vi "setMode.vi"(8 "error in (no error)":errorcluster, 10 "mode":enum16{"current", "voltage"}[](array[ring]), 11 "ethernetSupply in":refnum<class "ethernetSupply.lvclass">) -> (0 "error out":errorcluster, 3 "ethernetSupply out":refnum<class "ethernetSupply.lvclass">)   [LabVIEW 2011, in "Tools.lvlib" / "DatabaseHelpers.lvlib" / "ethernetSupply.lvclass"]
uses:
  ethernetSupply.lvclass
  ethernetSupply.lvclass/ethernetSupply.ctl
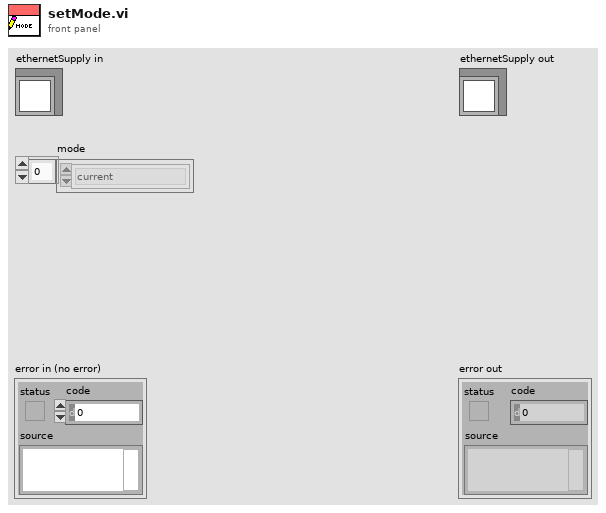
[diagram p1: front panel]
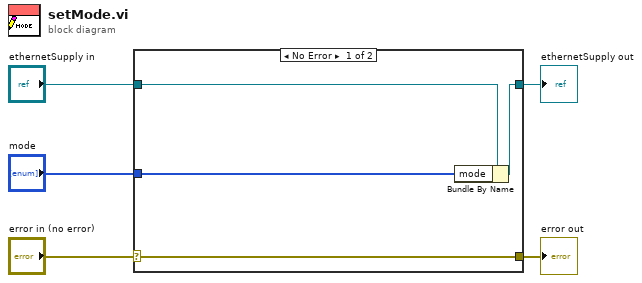
[diagram p0: block diagram]
diagram:
  n1 = case shown="No Error" "error in (no error)" {
    selector: "error in (no error)" -> [w9 w10]
    tunnel: [w9 w10] -> w4
    tunnel: [w7 w11] -> w2
    tunnel: "ethernetSupply in" -> [w8 w11]
    tunnel: "mode" -> [w6 _]
    frame No Error {
      n2 = Bundle By Name(cluster=w8, "mode"=w6) -> (w7:refnum<class "ethernetSupply.lvclass">)
    }
    frame Error {
    }
  }
  "error out" <- w4
  "ethernetSupply out" <- w2
